vi "P-DB.vi"(1 "Setpoint":dbl, 2 "Measured":dbl, 4 "Accepted error":dbl, 5 "Output":dbl) -> (0 "Output":dbl)   [LabVIEW 2014]
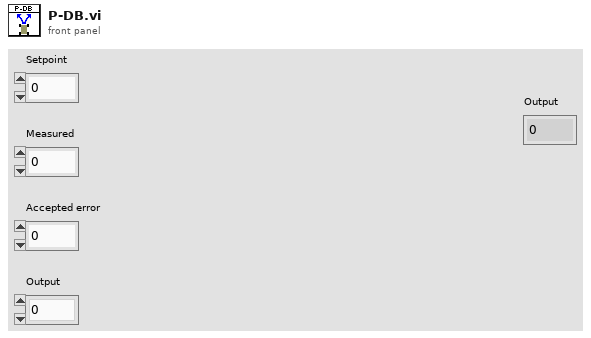
[diagram p1: front panel]
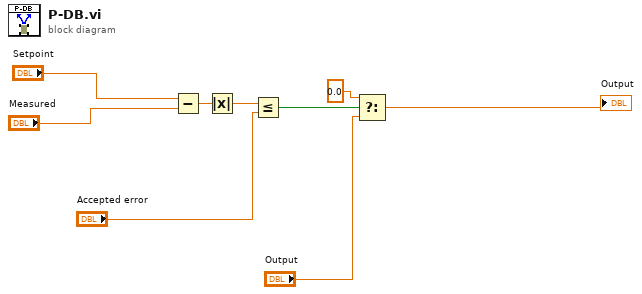
[diagram p0: block diagram]
diagram:
  n1 = Subtract(x="Setpoint", y="Measured") -> (x-y=w7:dbl)
  n2 = Absolute Value(x=w7) -> (abs(x)=w6:dbl)
  n3 = Less Or Equal?(x=w6, y="Accepted error") -> (x <= y?=w4:bool)
  n4 = Select(t=0.0, s=w4, f="Output") -> (s? t:f=→"Output":dbl)
